vi "UHR-Fleezers Control (host) - Lorentz v5.vi"() -> ()   [LabVIEW 2014] (continued)
            n3482 = property on="All FB On/Off" class="Bool (strict)"("Val(Sgnl)"=FALSE) -> ()  [unwired: 2 in, 2 out]
          }
        }
      }
    }
    n3483 = flat-sequence "To save data" {
      tunnel: [w5298] -> w4515
      tunnel: [w5299] -> w4514
      tunnel: w4477 -> [w5292]
      tunnel: w4206 -> [w5296]
      tunnel: ["Save Calibration"] -> w4489
      tunnel: w4236 -> [w5295]
      tunnel: [w5288] -> w4486
      tunnel: [w5285] -> w4485
      tunnel: [w5282] -> w4484
      tunnel: w4476 -> [w5284]
      tunnel: w4172 -> [w5278]
      tunnel: [w5278] -> w4440
      tunnel: ["Start Saving"] -> w4420
      tunnel: [w5273] -> w4369
      tunnel: [w5272] -> w4368
      tunnel: [w5269] -> w4270
      tunnel: [w5265] -> w4258
      tunnel: w4515 -> [w5610]
      tunnel: w4514 -> [w5609]
      tunnel: w4237 -> [w5608]
      tunnel: w4489 -> [w5607]
      tunnel: w4486 -> [w5605]
      tunnel: w4485 -> [w5604]
      tunnel: w4484 -> [w5603]
      tunnel: w4229 -> [w5602]
      tunnel: w4235 -> [w5601]
      tunnel: w4440 -> [w5600]
      tunnel: w4420 -> [w5599]
      tunnel: w4277 -> [w5598]
      tunnel: w4319 -> [w5597]
      tunnel: w4369 -> [w5596]
      tunnel: w4368 -> [w5595]
      tunnel: w4367 -> [w5594]
      tunnel: w4178 -> [w5593]
      tunnel: w4234 -> [w5592]
      tunnel: w4270 -> [w5591]
      tunnel: w4258 -> [w5590]
      frame #0 {
        # "Changed by Ronen - we don't have a database so we disabled this"
        n3484 = Or(x="Save N Sets", y="Start Saving") -> (x .or. y?=w5279:bool)
        n3485 = To Double Precision Float(number=w5295) -> (double precision float=w5289:dbl)
        n3486 = Build Array(w5279, "Save Calibration", w5292, w5284, "Flow Cal") -> (w5294:bool[])
        n3487 = Compound Arithmetic op=OR("Save Calibration", w5292, w5279, w5284, "Flow Cal") -> (w5297:bool)
        n3488 = Boolean Array To Number(Boolean array=w5294) -> (number=w5291:u32)
        n3489 = feedback #21(FALSE ("Save APD Data\nwith Trap Data")) -> (w5274:bool)
        n3490 = feedback #22(refnum<k0> refnum) -> (w5300:refnum<file>)
        n3491 = feedback #23(FALSE ("Save APD Data\nwith Trap Data")) -> (w5283:bool)
        n3492 = feedback #24(0) -> (w5302:i32)
        n3493 = feedback #25() -> (w5290:u32)  [unwired: 1 out]
        n3494 = feedback #26(refnum<k0> refnum) -> (w5270:refnum<file>)
        n3495 = feedback #27(refnum<k0> refnum) -> (w5276:refnum<file>)
        n3496 = feedback #28(refnum<k0> refnum) -> (w5266:refnum<file>)
        n3497 = feedback #29(refnum<k0> refnum) -> (w5286:refnum<file>)
        n3498 = case shown="True" w5297 {
          tunnel: [w5311 1] -> w5298
          tunnel: w5302 -> [w5313 _]
          tunnel: [w5312 w5345] -> w5299
          tunnel: w5300 -> [w5312 _]
          tunnel: w5296 -> [_ w5363]
          tunnel: w5289 -> [_ w5361]
          tunnel: w5291 -> [_ w5364]
          tunnel: [w5310 w5344] -> w5288
          tunnel: w5290 -> [w5310 _]
          tunnel: [w5309 w5342] -> w5285
          tunnel: w5286 -> [w5309 _]
          tunnel: [w5308 w5341] -> w5282
          tunnel: w5283 -> [w5308 _]
          tunnel: "Start Saving" -> [_ w5339]
          tunnel: w5278 -> [_ w5338]
          tunnel: [w5307 w5331] -> w5272
          tunnel: w5276 -> [w5307 _]
          tunnel: [w5306 w5330] -> w5273
          tunnel: w5274 -> [w5306 _]
          tunnel: [w5305 w5316] -> w5269
          tunnel: w5270 -> [w5305 _]
          tunnel: [w5304 w5314] -> w5265
          tunnel: w5266 -> [w5304 _]
          frame False {
            n3499 = Increment(x=w5313) -> (x+1=w5311:i32)
          }
          frame True {
            w5315 = FALSE ("Start Saving")
            w5340 = 10.0  # File Version
            w5347 = FALSE ("prepend array or string size? (T)")
            w5346 = T44."big-endian, network order" ("byte order (0:big-endian, network order)")
            # "Ronen Changed the create file - changed data folder to c:\\Data"
            # "Save trap position\ndata"
            n3500 = Array Size(array=w5338) -> (size(s)=w5337:i32)
            n3501 = To Double Precision Float(number=w5337) -> (double precision float=w5336:dbl)
            n3502 = local read "BD 1 Frequency 1 (MHz)"() -> (w5360:dbl)
            n3503 = local read "BD 2 Frequency 1 (MHz)"() -> (w5359:dbl)
            n3504 = local read "BD 1 Frequency 2 (MHz)"() -> (w5358:dbl)
            n3505 = local read "BD 2 Frequency 2 (MHz)"() -> (w5357:dbl)
            n3506 = local read "BD 1 Frequency 3 (MHz)"() -> (w5356:dbl)
            n3507 = local read "BD 2 Frequency 3 (MHz)"() -> (w5355:dbl)
            n3508 = local write "Flow Cal"(w5315) -> ()
            n3509 = local write "Save Calibration"(w5315) -> ()
            n3510 = local write "Start Saving"(w5315) -> ()
            n3511 = Build Array("Save APD Data\nwith Trap Data", "Save Trap Pos. Data") -> (w5333:bool[])
            n3512 = Boolean Array To Number(Boolean array=w5333) -> (number=w5332:u32)
            n3513 = Build Array(w5360, w5359, w5358, w5357, w5356, w5355) -> (w5354:dbl[])
            n3514 = case shown="16" w5364 {
              tunnel: w5363 -> [w5464 w5491 w5507 w5545 w5582]
              tunnel: w5336 -> [w5469 w5498 w5527 w5564 w5587]
              tunnel: w5361 -> [w5468 w5497 w5526 w5563 w5586]
              tunnel: [w5465 w5493 w5518 w5555 w5583] -> w5352
              tunnel: [w5456 "Cal sets to save" w5508 w5546 w5569] -> w5344
              tunnel: w5354 -> [w5466 w5494 w5520 w5557 w5584]
              tunnel: "Save APD Data\nwith Trap Data" -> [w5463 w5480 w5504 w5543 w5581]
              tunnel: [w5463 w5478 w5504 w5543 w5581] -> w5341
              tunnel: w5340 -> [w5459 w5487 w5502 w5541 w5577]
              tunnel: w5339 -> [w5458 _ _ _ _]
              tunnel: [w5449 w5486 w5501 w5531 w5576] -> w5330
              tunnel: "Save Trap Pos. Data" -> [w5449 w5485 w5501 w5531 w5576]
              tunnel: w5332 -> [w5448 w5484 w5500 w5530 w5575]
              frame 1, Default {
                # "timeseries"
                n3515 = case shown="True" "Profile" {
                  tunnel: [w5472 w5476] -> w5453
                  tunnel: [w5472 w5475] -> w5452
                  tunnel: [w5472 w5474] -> w5451
                  tunnel: [w5472 w5473] -> w5450
                  frame False {
                    w5472 = 0.0 ("f")
                  }
                  frame True {
                    n3516 = local read "Current Position"() -> (w5477:cluster{dbl, dbl, dbl})
                    n3517 = local read "Y change (mm)"() -> (w5473:dbl)
                    n3518 = Unbundle(w5477) -> (w5476:dbl, w5475:dbl, w5474:dbl)
                  }
                }
                n3519 = local read "Save ave N"() -> (w5471:dbl)
                n3520 = Multiply(x=w5471, y=w5464) -> (x*y=w5470:dbl)
                n3521 = To Double Precision Float(number=w5448) -> (double precision float=w5462:dbl)
                n3522 = Build Array(w5459, w5464, w5470, w5469, w5468, 0.0 ("f")) -> (w5467:dbl[])
                n3523 = Build Array(w5462, w5453, w5452, w5451, w5450) -> (w5460:dbl[])
                n3524 = Select(t=u32 4000000000, s=w5458, f="N sets to save") -> (s? t:f=w5456:u32)
                n3525 = Build Array (concatenate)(w5467, w5466, w5460) -> (w5465:dbl[])
              }
              frame 2 {
                w5489 = 0.0 ("f")
                w5479 = FALSE ("Save APD Data\nwith Trap Data")
                # "For diagnostics save trap position\ndata during cal"
                # "calibration"
                n3526 = Boolean To (0,1)(Boolean=w5479) -> (0, 1=w5483:i16)
                n3527 = Select(t=w5480, s="Save trap pos with cal", f=w5479) -> (s? t:f=w5478:bool)
                n3528 = Select(t=w5485, s="Save trap pos with cal", f=w5479) -> (s? t:f=w5486:bool)
                n3529 = Select(t=w5484, s="Save trap pos with cal", f=w5483) -> (s? t:f=w5482:u32)
                n3530 = To Double Precision Float(number=w5482) -> (double precision float=w5490:dbl)
                n3531 = Build Array(w5487, w5491, w5491, w5498, w5497, 1.0 ("t")) -> (w5495:dbl[])
                n3532 = Build Array(w5490, w5489, w5489, w5489, w5489) -> (w5488:dbl[])
                n3533 = Build Array (concatenate)(w5495, w5494, w5488) -> (w5493:dbl[])
                "Calibrating Trap..." <- TRUE ("Calibrating...")
              }
              frame 4 {
                w5505 = 0.0 ("f")
                # "scan dir (x/y = 0/1)"
                # "cycles/step"
                # "n scans (f/b)"
                # "steps"
                # "freq. range"
                # "AOD raster scan"
                n3534 = local read "Number of F/B Scans (AOD)"() -> (w5512:u16)
                n3535 = local read "Cycles/step (AOD)"() -> (w5514:u64)
                n3536 = local read "Scan Range (MHz)"() -> (w5517:dbl)
                n3537 = local read "Scan steps (AOD)"() -> (w5516:u64)
                n3538 = local read "Scan BD"() -> (w5524:bool)
                n3539 = local read "Save ave N"() -> (w5529:dbl)
                n3540 = Boolean To (0,1)(Boolean=w5524) -> (0, 1=w5523:i16)
                n3541 = To Double Precision Float(number=w5512) -> (double precision float=w5511:dbl)
                n3542 = To Double Precision Float(number=w5516) -> (double precision float=w5515:dbl)
                n3543 = To Double Precision Float(number=w5514) -> (double precision float=w5513:dbl)
                n3544 = To Double Precision Float(number=w5523) -> (double precision float=w5522:dbl)
                n3545 = Multiply(x=w5529, y=w5507) -> (x*y=w5528:dbl)
                n3546 = To Double Precision Float(number=w5500) -> (double precision float=w5506:dbl)
                n3547 = Build Array(w5506, w5505, w5505, w5505, w5505) -> (w5503:dbl[])
                n3548 = local read "N sets should be saved"() -> (w5509:dbl)
                n3549 = Build Array(w5522, w5517, w5515, w5513, w5511) -> (w5519:dbl[])
                n3550 = Build Array(w5502, w5507, w5528, w5527, w5526, 2.0 ("t")) -> (w5521:dbl[])
                n3551 = Round Toward +Infinity(x=w5509) -> (ceil(x): smallest int >= x=w5510:dbl)
                n3552 = Build Array (concatenate)(w5521, w5520, w5503, w5519) -> (w5518:dbl[])
                n3553 = To Unsigned Long Integer(number=w5510) -> (unsigned 32bit integer=w5508:u32)
              }
              frame 8 {
                w5538 = 0.0 ("f")
                # "MCL raster scan"
                n3554 = local read "Number of scans (MCL)"() -> (w5533:u64)
                n3555 = local read "2D or 1D Scan"() -> (w5535:bool)
                n3556 = local read "Scan lines (y)"() -> (w5532:u64)
                n3557 = local read "Scan Range (V)\n(of steps)"() -> (w5554:dbl)
                n3558 = local read "Fast Scan Dir"() -> (w5561:bool)
                n3559 = local read "Cycles/step (MCL)"() -> (w5551:u64)
                n3560 = local read "Scan steps (MCL)"() -> (w5553:u64)
                n3561 = Select(t=w5532, s=w5535, f=w5533) -> (s? t:f=w5534:u64)
                n3562 = Boolean To (0,1)(Boolean=w5535) -> (0, 1=w5537:i16)
                n3563 = local read "Save ave N"() -> (w5566:dbl)
                n3564 = local read "Initial X"() -> (w5540:dbl)
                n3565 = local read "Initial Y"() -> (w5539:dbl)
                n3566 = To Double Precision Float(number=w5537) -> (double precision float=w5536:dbl)
                n3567 = Boolean To (0,1)(Boolean=w5561) -> (0, 1=w5560:i16)
                n3568 = To Double Precision Float(number=w5534) -> (double precision float=w5549:dbl)
                n3569 = To Double Precision Float(number=w5553) -> (double precision float=w5552:dbl)
                n3570 = To Double Precision Float(number=w5551) -> (double precision float=w5550:dbl)
                n3571 = To Double Precision Float(number=w5560) -> (double precision float=w5559:dbl)
                n3572 = Multiply(x=w5566, y=w5545) -> (x*y=w5565:dbl)
                n3573 = To Double Precision Float(number=w5530) -> (double precision float=w5544:dbl)
                n3574 = local read "N sets should be saved (MCL)"() -> (w5547:dbl)
                n3575 = Build Array(w5544, w5536, w5538, w5538, w5538) -> (w5542:dbl[])
                n3576 = Build Array(w5559, w5554, w5552, w5550, w5549, w5540, w5539) -> (w5556:dbl[])
                n3577 = Build Array(w5541, w5545, w5565, w5564, w5563, 3.0 ("t")) -> (w5558:dbl[])
                n3578 = Round Toward +Infinity(x=w5547) -> (ceil(x): smallest int >= x=w5548:dbl)
                n3579 = Build Array (concatenate)(w5558, w5557, w5542, w5556) -> (w5555:dbl[])
                n3580 = To Unsigned Long Integer(number=w5548) -> (unsigned 32bit integer=w5546:u32)
              }
              frame 16 {
                w5568 = 0.0
                # "Flow calibration - added by Ronen: Number\nof saved sets is distance (1 mm) divided by \nspeed +1.5 spare second divided by the time of\nset measurement, 0.2 sec for 2 set interlace"
                # "timeseries"
                n3581 = local read "Save ave N"() -> (w5589:dbl)
                n3582 = Reciprocal(x=0.0) -> (1/x=w5574:dbl)
                n3583 = Add(x=w5574, y=1.5) -> (x+y=w5572:dbl)
                n3584 = Multiply(x=w5589, y=w5582) -> (x*y=w5588:dbl)
                n3585 = Divide(x=w5572, y=0.2) -> (x/y=w5570:dbl)
                n3586 = To Double Precision Float(number=w5575) -> (double precision float=w5580:dbl)
                n3587 = To Unsigned Long Integer(number=w5570) -> (unsigned 32bit integer=w5569:u32)
                n3588 = Build Array(w5577, w5582, w5588, w5587, w5586, 4.0 ("f")) -> (w5585:dbl[])
                n3589 = Build Array(w5580, w5568, w5568, w5568, w5568) -> (w5578:dbl[])
                n3590 = Build Array (concatenate)(w5585, w5584, w5578) -> (w5583:dbl[])
              }
            }
            n3591 = local read "Index"() -> (w5369:dbl)
            n3592 = call "Create new save file.vi"("Insert"="", "Ext"=".dat", "Index In"=w5369) -> ("Path Out"=w5318:path, "Index Out"=w5343:dbl)
            n3593 = local write "Save file name"(w5318) -> ()
            n3594 = local write "Index"(w5343) -> ()
            n3595 = local write "Save index"(w5343) -> ()
            n3596 = case shown="True" "Save Event Log?" {
              tunnel: w5318 -> [_ w5383]
              tunnel: [refnum<k0> refnum w5382] -> w5316
              frame False {
              }
              frame True {
                (unwired) FALSE ("prepend array or string size? (T)")
                n3597 = Path To String(path=w5383) -> (string=w5394:string)
                n3598 = String Length(string=w5394) -> (length=w5393:i32)
                n3599 = Subtract(x=w5393, y=4) -> (x-y=w5391:i32)
                n3600 = String Subset(string=w5394, length (rest)=w5391) -> (substring=w5390:string)  [unwired: 1 out]
                n3601 = Concatenate Strings(w5390, "_log.txt" ("string")) -> (w5388:string)
                n3602 = String To Path(string=w5388) -> (path=w5384:path)
                n3603 = Open/Create/Replace File(file path (use dialog)=w5384, operation (0:open)=T43."create", access (0:read/write)=enum16{"read/write", "read-only", "write-only"}."write-only") -> (refnum out=w5385:refnum<file>)  [unwired: 1 in, 4 out]
                n3604 = Deny Access(7:w5385) -> (3:w5382:refnum<file>)  [unwired: 1 in, 2 out]
                n3605 = call "write to event log.vi"("log file ref"=w5382, "time"=0.0, "input string"="start log") -> ()  [unwired: 8 in]
              }
            }
            "log file ref" <- w5316
            n3606 = Array Size(array=w5352) -> (size(s)=w5353:i32)
            n3607 = Open/Create/Replace File(file path (use dialog)=w5318, operation (0:open)=T43."create", access (0:read/write)=enum16{"read/write", "read-only", "write-only"}."write-only") -> (refnum out=w5366:refnum<file>)  [unwired: 1 in, 4 out]
            n3608 = local write "Saving..."(TRUE ("Saving...")) -> ()
            n3609 = To Double Precision Float(number=w5353) -> (double precision float=w5351:dbl)
            n3610 = String Length(string="Comment (data description)") -> (length=w5350:i32)
            n3611 = To Double Precision Float(number=w5350) -> (double precision float=w5349:dbl)
            n3612 = Deny Access(7:w5366) -> (3:w5365:refnum<file>)  [unwired: 1 in, 2 out]
            n3613 = Build Array (concatenate)(w5351, w5352, w5349) -> (w5328:dbl[])
            n3614 = case "If fluorescence data to be saved" shown="True" w5341 {
              tunnel: w5318 -> [_ w5447]
              tunnel: [w5417 w5430] -> w5342
              tunnel: [w5417 w5418] -> w5314
              frame False {
                w5417 = refnum<k0> refnum
              }
              frame True {
                w5429 = 0.0
                w5422 = T43."create" ("operation (0:open)")
                w5423 = enum16{"read/write", "read-only", "write-only"}."write-only" ("access (0:read/write)")
                n3615 = local read "APD Integration Time (s)"() -> (w5435:dbl)
                n3616 = local read "N APD Samp/step"() -> (w5428:dbl)
                n3617 = local read "Number of APDs"() -> (w5427:u8)
                n3618 = Path To String(path=w5447) -> (string=w5446:string)
                n3619 = String Length(string=w5446) -> (length=w5445:i32)
                n3620 = Subtract(x=w5445, y=4) -> (x-y=w5443:i32)
                n3621 = String Subset(string=w5446, length (rest)=w5443) -> (substring=w5426:string)  [unwired: 1 out]
                n3622 = Build Array(w5435, w5428, w5427, w5429, w5429, w5429, w5429, w5429) -> (w5432:dbl[])
                n3623 = Concatenate Strings(w5426, "_green.dat") -> (w5424:string)
                n3624 = Concatenate Strings(w5426, "_fl.dat" ("string")) -> (w5441:string)
                n3625 = Array Size(array=w5432) -> (size(s)=w5434:i32)
                n3626 = String To Path(string=w5441) -> (path=w5439:path)
                n3627 = Open/Create/Replace File(file path (use dialog)=w5439, operation (0:open)=w5422, access (0:read/write)=w5423) -> (refnum out=w5440:refnum<file>)  [unwired: 1 in, 4 out]
                n3628 = Deny Access(7:w5440) -> (3:w5436:refnum<file>)  [unwired: 1 in, 2 out]
                n3629 = String To Path(string=w5424) -> (path=w5421:path)
                n3630 = To Double Precision Float(number=w5434) -> (double precision float=w5433:dbl)
                n3631 = Build Array (concatenate)(w5433, w5432) -> (w5431:dbl[])
                n3632 = Write to Binary File(file (use dialog)=w5436, data=w5431, 5:FALSE ("prepend array or string size? (T)"), 9:T44."big-endian, network order" ("byte order (0:big-endian, network order)")) -> (refnum out=w5430:refnum<file>)  [unwired: 1 in, 3 out]
                n3633 = Open/Create/Replace File(file path (use dialog)=w5421, operation (0:open)=w5422, access (0:read/write)=w5423) -> (refnum out=w5419:refnum<file>, error out=w5420:errorcluster)  [unwired: 3 in, 1 out]
                n3634 = Deny Access(4:w5420, 7:w5419) -> (3:w5418:refnum<file>)  [unwired: 1 in, 1 out]
              }
            }
            n3635 = case shown="True" w5330 {
              tunnel: w5318 -> [_ w5402]
              tunnel: [refnum<k0> refnum w5401] -> w5331
              frame False {
              }
              frame True {
                w5397 = 0.0 ("element")
                n3636 = Path To String(path=w5402) -> (string=w5416:string)
                n3637 = Build Array(w5397, w5397, w5397, w5397, w5397, w5397, w5397, w5397) -> (w5398:dbl[])
                n3638 = String Length(string=w5416) -> (length=w5415:i32)
                n3639 = Subtract(x=w5415, y=4) -> (x-y=w5413:i32)
                n3640 = Array Size(array=w5398) -> (size(s)=w5400:i32)
                n3641 = String Subset(string=w5416, length (rest)=w5413) -> (substring=w5412:string)  [unwired: 1 out]
                n3642 = To Double Precision Float(number=w5400) -> (double precision float=w5399:dbl)
                n3643 = Concatenate Strings(w5412, "_pos.dat" ("string")) -> (w5410:string)
                n3644 = Build Array (concatenate)(w5399, w5398) -> (w5396:dbl[])
                n3645 = String To Path(string=w5410) -> (path=w5406:path)
                n3646 = Open/Create/Replace File(file path (use dialog)=w5406, operation (0:open)=T43."create", access (0:read/write)=enum16{"read/write", "read-only", "write-only"}."write-only") -> (refnum out=w5407:refnum<file>)  [unwired: 1 in, 4 out]
                n3647 = Deny Access(7:w5407) -> (3:w5403:refnum<file>)  [unwired: 1 in, 2 out]
                n3648 = Write to Binary File(file (use dialog)=w5403, data=w5396, 5:FALSE ("prepend array or string size? (T)"), 9:T44."big-endian, network order" ("byte order (0:big-endian, network order)")) -> (refnum out=w5401:refnum<file>)  [unwired: 1 in, 3 out]
              }
            }
            n3649 = Write to Binary File(file (use dialog)=w5365, data=w5328, 5:w5347, 9:w5346) -> (refnum out=w5348:refnum<file>)  [unwired: 1 in, 3 out]
            n3650 = Write to Binary File(file (use dialog)=w5348, data="Comment (data description)", 5:w5347, 9:w5346) -> (refnum out=w5345:refnum<file>)  [unwired: 1 in, 3 out]
            n3651 = local read "connection reference"() -> (w5329:T24)
            n3652 = Bundle("Comment (data description)"="Comment (data description)", "Channel 1 Buffer"="Channel 1 Buffer", "Channel 2 Buffer"="Channel 2 Buffer", "Channel 3 Buffer"="Channel 3 Buffer", "Title"="Title", "DNA Construct"="DNA Construct", "Bead diameter"="Bead diameter", "Name"="Name") -> (w5319:T63)  [unwired: 1 in]
            n3653 = disable-structure shown="Disabled" {
              disable-tunnel: w5329 -> [w5377 _]
              disable-tunnel: w5328 -> [w5375 _]
              disable-tunnel: w5319 -> [w5374 _]
              disable-tunnel: w5318 -> [w5373 _]
              frame Disabled {
                n3654 = call "MattFileCreator-v9.vi"("Comments"=w5374, "Input Array"=w5375, "File path"=w5373, "table"="labview", "connection reference"=w5377) -> ("connection reference out"=w5376:T24)  [unwired: 5 in, 1 out]
                n3655 = local write "connection reference"(w5376) -> ()
              }
              frame Enabled {
              }
            }
          }
        }
        n3656 = feedback-in #21(w5273) -> ()
        n3657 = feedback-in #22(w5299) -> ()
        n3658 = feedback-in #23(w5282) -> ()
        n3659 = feedback-in #24(w5298) -> ()
        n3660 = feedback-in #25(w5288) -> ()
        n3661 = feedback-in #26(w5269) -> ()
        n3662 = feedback-in #27(w5272) -> ()
        n3663 = feedback-in #28(w5265) -> ()
        n3664 = feedback-in #29(w5285) -> ()
      }
      frame #1 {
        n3665 = local read "Saving..."() -> (w5606:bool)
        n3666 = case shown="True" w5606 {
          tunnel: w5610 -> [_ w5624]
          tunnel: w5609 -> [_ w5638]
          tunnel: w5608 -> [_ w5634]
          tunnel: w5607 -> [_ w5633]
          tunnel: w5605 -> [_ w5632]
          tunnel: w5604 -> [_ w5627]
          tunnel: w5603 -> [_ w5626]
          tunnel: w5602 -> [_ w5625]
          tunnel: w5601 -> [_ w5623]
          tunnel: w5600 -> [_ w5621]
          tunnel: w5599 -> [_ w5620]
          tunnel: w5598 -> [_ w5619]
          tunnel: w5597 -> [_ w5618]
          tunnel: w5596 -> [_ w5617]
          tunnel: w5595 -> [_ w5616]
          tunnel: w5594 -> [_ w5615]
          tunnel: w5593 -> [_ w5614]
          tunnel: w5592 -> [_ w5613]
          tunnel: w5591 -> [_ w5612]
          tunnel: w5590 -> [_ w5611]
          frame False {
          }
          frame True {
            n3667 = Multiply(x=w5624, y=w5623) -> (x*y=→"Time (s)":dbl)
            n3668 = Less Or Equal?(x=w5624, y=w5632) -> (x <= y?=w5636:bool)
            n3669 = Compound Arithmetic op=OR("Stop Saving", "Abort save 2") -> (w5628:bool)
            n3670 = Not(x=w5628) -> (.not. x?=w5637:bool)
            n3671 = And(x=w5636, y=w5637) -> (x .and. y?=w5635:bool)
            n3672 = case shown="True" w5635 {
              tunnel: w5638 -> [w5648 w5749]
              tunnel: [0.0 w5752] -> w5631
              tunnel: w5624 -> [_ w5750]
              tunnel: w5632 -> [_ w5751]
              tunnel: w5634 -> [_ w5746]
              tunnel: w5633 -> [_ _]
              tunnel: w5627 -> [w5646 w5739]
              tunnel: w5626 -> [w5645 w5740]
              tunnel: w5625 -> [_ w5738]
              tunnel: w5621 -> [_ w5737]
              tunnel: w5620 -> [_ w5655]
              tunnel: w5619 -> [_ w5730]
              tunnel: w5618 -> [_ w5677]
              tunnel: w5617 -> [w5642 w5694]
              tunnel: w5616 -> [w5643 w5693]
              tunnel: w5615 -> [_ w5690]
              tunnel: w5614 -> [_ w5688]
              tunnel: w5613 -> [_ w5654]
              tunnel: w5612 -> [w5641 _]
              tunnel: w5611 -> [w5639 w5653]
              frame False {
                w5644 = FALSE
                n3673 = Close File(refnum=w5648) -> ()  [unwired: 1 in, 2 out]
                n3674 = case shown="True" w5645 {
                  tunnel: w5646 -> [_ w5652]
                  tunnel: w5639 -> [_ w5651]
                  frame False {
                  }
                  frame True {
                    n3675 = Close File(refnum=w5652) -> ()  [unwired: 1 in, 2 out]
                    n3676 = Close File(refnum=w5651) -> ()  [unwired: 1 in, 2 out]
                  }
                }
                n3677 = case shown="True" w5642 {
                  tunnel: w5643 -> [_ w5650]
                  frame False {
                  }
                  frame True {
                    n3678 = Close File(refnum=w5650) -> ()  [unwired: 1 in, 2 out]
                  }
                }
                n3679 = local read "Save Event Log?"() -> (w5640:bool)
                n3680 = case shown="True" w5640 {
                  tunnel: w5641 -> [_ w5649]
                  frame False {
                  }
                  frame True {
                    n3681 = Close File(refnum=w5649) -> ()  [unwired: 1 in, 2 out]
                  }
                }
                n3682 = local write "Raster Scanning..."(w5644) -> ()
                n3683 = local write "Calibrating Trap..."(w5644) -> ()
                n3684 = call <vilib>:"Beep.vi"() -> ()  [unwired: 3 in, 9 out]
                n3685 = local write "Stop Saving"(w5644) -> ()
                "Saving..." <- w5644
              }
              frame True {
                n3686 = local read "Calibrating Trap..."() -> (w5741:bool)
                n3687 = case "Write fl. data" shown="True" w5740 {
                  tunnel: w5739 -> [_ w5782]
                  tunnel: w5738 -> [_ w5781]
                  tunnel: w5653 -> [_ w5775]
                  frame False {
                  }
                  frame True {
                    w5774 = FALSE ("prepend array or string size? (T)")
                    w5776 = T44."big-endian, network order" ("byte order (0:big-endian, network order)")
                    n3688 = property on="Green Laser ON" class="Bool (strict)"() -> ("Value"=w5780:bool)  [unwired: 2 in, 2 out]
                    n3689 = property on="Green Intensity % (FB OFF)" class="DigNum (strict)"() -> ("Value"=w5779:dbl)  [unwired: 2 in, 2 out]
                    n3690 = Boolean To (0,1)(Boolean=w5780) -> (0, 1=w5778:i16)
                    n3691 = Multiply(x=w5778, y=w5779) -> (x*y=w5777:dbl)
                    n3692 = Write to Binary File(file (use dialog)=w5782, data=w5781, 5:w5774, 9:w5776) -> ()  [unwired: 1 in, 4 out]
                    n3693 = Write to Binary File(file (use dialog)=w5775, data=w5777, 5:w5774, 9:w5776) -> ()  [unwired: 2 in, 3 out]
                  }
                }
                n3694 = Greater?(x="Save ave N", y=1.0) -> (0:w5744:bool)
                n3695 = Not(x=w5741) -> (.not. x?=w5743:bool)
                n3696 = And(x=w5743, y=w5744) -> (x .and. y?=w5691:bool)
                n3697 = case shown="True" w5691 {
                  tunnel: w5690 -> [w5755 w5766]
                  tunnel: [w5755 w5758] -> w5689
                  tunnel: "Save ave N" -> [_ w5759]
                  frame False {
                  }
                  frame True {
                    w5756 = 2 ("dimension size")
                    n3698 = Array Size(array=w5766) -> (size(s)=w5760:i32)
                    n3699 = Divide(x=w5760, y=w5756) -> (x/y=w5764:dbl)
                    n3700 = Reshape Array(w5766, w5764, w5756) -> (w5765:u64[][])
                    n3701 = Transpose 2D Array(2D array=w5765) -> (transposed array=w5763:u64[][])
                    n3702 = for {
                      tunnel: w5763 -> [w5768] mode=indexing
                      tunnel: [w5767] -> w5757 mode=indexing
                      tunnel: w5759 -> [w5769]
                      workers-P: _ -> [_]
                      n3703 = call "downsample 1D array - U64.vi"("Ave N"=w5769, "Array In"=w5768) -> ("Array Out"=w5767:u64[])  [unwired: 1 in]
                    }
                    n3704 = Transpose 2D Array(2D array=w5757) -> (transposed array=w5762:u64[][])
                    n3705 = Divide(x=w5760, y=w5759) -> (x/y=w5761:dbl)
                    n3706 = Reshape Array(w5762, w5761) -> (w5758:u64[])
                  }
                }
                n3707 = case shown="True" w5691 {
                  tunnel: w5746 -> [w5783 w5795]
                  tunnel: [w5783 w5787] -> w5742
                  tunnel: "Save ave N" -> [_ w5788]
                  tunnel: w5737 -> [_ w5786]
                  frame False {
                  }
                  frame True {
                    n3708 = Array Size(array=w5795) -> (size(s)=w5789:i32)
                    n3709 = Array Size(array=w5786) -> (size(s)=w5785:i32)
                    n3710 = Divide(x=w5789, y=w5785) -> (x/y=w5793:dbl)
                    n3711 = Reshape Array(w5795, w5793, w5785) -> (w5794:i16[][])
                    n3712 = Transpose 2D Array(2D array=w5794) -> (transposed array=w5792:i16[][])
                    n3713 = for {
                      tunnel: w5792 -> [w5798] mode=indexing
                      tunnel: [w5797] -> w5784 mode=indexing
                      tunnel: w5788 -> [w5796]
                      workers-P: _ -> [_]
                      n3714 = call "downsample 1D array - I16 to F32.vi"("Ave N"=w5796, "Array In"=w5798) -> ("Array Out"=w5797:sgl[])  [unwired: 1 in]
                    }
                    n3715 = Transpose 2D Array(2D array=w5784) -> (transposed array=w5791:sgl[][])
                    n3716 = Divide(x=w5789, y=w5788) -> (x/y=w5790:dbl)
                    n3717 = Reshape Array(w5791, w5790) -> (w5787:sgl[])
                  }
                }
                n3718 = Index Array(array=w5677, index=2) -> (element=w5678:waveform(dbl))
                n3719 = Index Array(array=w5677, index=1) -> (element=w5711:waveform(dbl))
                n3720 = Index Array(array=w5677, index=0) -> (element=w5713:waveform(dbl))
                n3721 = Unbundle By Name(w5678) -> ("Y"=w5680:dbl[])
                n3722 = Unbundle By Name(w5711) -> ("Y"=w5715:dbl[])
                n3723 = Unbundle By Name(w5713) -> ("Y"=w5723:dbl[])
                n3724 = case "Write trap pos. data" shown="True" w5694 {
                  tunnel: w5693 -> [_ w5771]
                  tunnel: w5689 -> [_ w5770]
                  frame False {
                  }
                  frame True {
                    n3725 = Write to Binary File(file (use dialog)=w5771, data=w5770, 5:FALSE ("prepend array or string size? (T)"), 9:T44."big-endian, network order" ("byte order (0:big-endian, network order)")) -> ()  [unwired: 1 in, 4 out]
                  }
                }
                n3726 = Write to Binary File(file (use dialog)=w5749, data=w5742, 5:FALSE ("prepend array or string size? (T)"), 9:T44."big-endian, network order" ("byte order (0:big-endian, network order)")) -> ()  [unwired: 1 in, 4 out]
                n3727 = feedback #30(w5680) -> (w5681:dbl[])
                n3728 = Build Array (concatenate)(w5681, w5680) -> (w5676:dbl[])
                n3729 = Select(t=w5680, s=w5655, f=w5676) -> (s? t:f=w5666:dbl[])
                n3730 = feedback-in #30(w5666) -> ()
                n3731 = feedback #31(w5715) -> (w5717:dbl[])
                n3732 = Build Array (concatenate)(w5717, w5715) -> (w5716:dbl[])
                n3733 = Select(t=w5715, s=w5655, f=w5716) -> (s? t:f=w5705:dbl[])
                n3734 = feedback-in #31(w5705) -> ()
                n3735 = feedback #32(w5723) -> (w5736:dbl[])
                n3736 = Build Array (concatenate)(w5736, w5723) -> (w5735:dbl[])
                n3737 = Select(t=w5723, s=w5655, f=w5735) -> (s? t:f=w5710:dbl[])
                n3738 = feedback-in #32(w5710) -> ()
                n3739 = Divide(x=w5750, y=w5751) -> (x/y=w5753:dbl)
                n3740 = Multiply(x=w5753, y=100.0) -> (x*y=w5752:dbl)
                n3741 = Build Array(w5710, w5705, w5666) -> (→"Saved APD":dbl[][])
                n3742 = Array Size(array=w5710) -> (size(s)=w5728:i32)
                n3743 = Unbundle By Name(w5730) -> ("Y"=w5734:dbl[])
                n3744 = Subtract(x=w5728, y="N pts to average") -> (x-y=w5663:i32)
                n3745 = Multiply(x="N pts to average", y=u16 2) -> (x*y=w5706:u16)
                n3746 = Subtract(x=w5728, y=w5706) -> (x-y=w5664:i32)
                n3747 = feedback #33(w5734) -> (w5733:dbl[])
                n3748 = Build Array (concatenate)(w5733, w5734) -> (w5732:dbl[])
                n3749 = Select(t=w5734, s=w5655, f=w5732) -> (s? t:f=w5731:dbl[])
                "Trap Delta Graph" <- w5731
                n3750 = feedback-in #33(w5731) -> ()
                n3751 = Array Subset(array=w5710, index=w5663, length="N pts to average") -> (w5727:dbl[])
                n3752 = Array Subset(array=w5710, index=w5664, length="N pts to average") -> (w5726:dbl[])
                n3753 = Array Subset(array=w5705, index=w5663, length="N pts to average") -> (w5708:dbl[])
                n3754 = Array Subset(array=w5705, index=w5664, length="N pts to average") -> (w5707:dbl[])
                n3755 = Array Subset(array=w5666, index=w5663, length="N pts to average") -> (w5675:dbl[])
                n3756 = Array Subset(array=w5666, index=w5664, length="N pts to average") -> (w5674:dbl[])
                n3757 = Index Array(array=w5688, index=0) -> (element=w5686:waveform(dbl))
                n3758 = call-poly <vilib>:"Mean.vi"("X"=w5727) -> ("mean"=w5725:dbl)  [unwired: 1 out]
                n3759 = call-poly <vilib>:"Mean.vi"("X"=w5708) -> ("mean"=w5704:dbl)  [unwired: 1 out]
                n3760 = call-poly <vilib>:"Mean.vi"("X"=w5726) -> ("mean"=w5724:dbl)  [unwired: 1 out]
                n3761 = call-poly <vilib>:"Mean.vi"("X"=w5707) -> ("mean"=w5703:dbl)  [unwired: 1 out]
                n3762 = call-poly <vilib>:"Mean.vi"("X"=w5675) -> ("mean"=w5673:dbl)  [unwired: 1 out]
                n3763 = call-poly <vilib>:"Mean.vi"("X"=w5674) -> ("mean"=w5672:dbl)  [unwired: 1 out]
                n3764 = Unbundle By Name(w5686) -> ("Y"=w5684:dbl[])
                n3765 = Subtract(x=w5704, y=w5703) -> (x-y=w5695:dbl)
                "Delta Fl. 2" <- w5695
                n3766 = Subtract(x=w5673, y=w5672) -> (x-y=w5667:dbl)
                "Delta Fl. 3" <- w5667
                n3767 = Subtract(x=w5725, y=w5724) -> (x-y=w5722:dbl)
                "Delta Fl. 1" <- w5722
                n3768 = feedback #34(w5684) -> (w5683:dbl[])
                n3769 = Build Array (concatenate)(w5683, w5684) -> (w5685:dbl[])
                n3770 = Initialize Array(w5722, 1 ("dimension size")) -> (w5719:dbl[])
                n3771 = Initialize Array(w5695, 1 ("dimension size")) -> (w5700:dbl[])
                n3772 = Initialize Array(w5667, 1 ("dimension size")) -> (w5669:dbl[])
                n3773 = Select(t=w5684, s=w5655, f=w5685) -> (s? t:f=w5682:dbl[])
                "Saved trap pos" <- w5682
                n3774 = feedback-in #34(w5682) -> ()
                n3775 = feedback #35(w5719) -> (w5720:dbl[])
                n3776 = Build Array (concatenate)(w5720, w5719) -> (w5718:dbl[])
                n3777 = feedback #36(w5700) -> (w5701:dbl[])
                n3778 = feedback #37(w5669) -> (w5670:dbl[])
                n3779 = Build Array (concatenate)(w5701, w5700) -> (w5699:dbl[])
                n3780 = Build Array (concatenate)(w5670, w5669) -> (w5668:dbl[])
                n3781 = Select(t=w5719, s=w5655, f=w5718) -> (s? t:f=w5698:dbl[])
                n3782 = feedback-in #35(w5698) -> ()
                n3783 = Select(t=w5700, s=w5655, f=w5699) -> (s? t:f=w5697:dbl[])
                n3784 = feedback-in #36(w5697) -> ()
                n3785 = Select(t=w5669, s=w5655, f=w5668) -> (s? t:f=w5662:dbl[])
                n3786 = feedback-in #37(w5662) -> ()
                n3787 = Build Array(w5698, w5697, w5662) -> (→"Save APD Deriv":dbl[][])
                n3788 = Index Array(array=w5654, index=15) -> (element=w5660:waveform(dbl))
                n3789 = Unbundle By Name(w5660) -> ("Y"=w5658:dbl[])
                n3790 = feedback #38(w5658) -> (w5657:dbl[])
                n3791 = Build Array (concatenate)(w5657, w5658) -> (w5659:dbl[])
                n3792 = Select(t=w5658, s=w5655, f=w5659) -> (s? t:f=w5656:dbl[])
                "Amp current" <- w5656
                n3793 = feedback-in #38(w5656) -> ()
              }
            }
            "Progress" <- w5631
            "Progress 2" <- w5631
          }
        }
      }
    }
    n3794 = local read "wait to reset values"() -> (w4499:bool)
    n3795 = Not(x=w4497) -> (.not. x?=w4500:bool)
    n3796 = And(x=w4500, y=w4499) -> (x .and. y?=w4501:bool)
    n3797 = case "Part of MCL raster scanning: returns to initial positions after scan done" shown="True" w4501 {
      tunnel: w4247 -> [w5094 w5101]
      tunnel: [w5094 w5100] -> w4503
      tunnel: w4348 -> [w5093 w5099]
      tunnel: [w5093 w5098] -> w4498
      frame False {
      }
      frame True {
        w5109 = 10.0 ("y")
        w5108 = 32767.0 ("y")
        # "to return scan values\nafter a synchronous \nAOM scan"
        n3798 = local read "AO2"() -> (w5102:dbl)
        n3799 = local read "AO1"() -> (w5103:dbl)
        n3800 = local write "wait to reset values"(FALSE ("wait to reset values")) -> ()
        n3801 = Multiply(x=w5103, y=w5108) -> (x*y=w5105:dbl)
        n3802 = Multiply(x=w5102, y=w5108) -> (x*y=w5107:dbl)
        n3803 = Divide(x=w5105, y=w5109) -> (x/y=w5104:dbl)
        n3804 = Divide(x=w5107, y=w5109) -> (x/y=w5106:dbl)
        n3805 = To Word Integer(number=w5104) -> (16bit integer=w5110:i16)
        n3806 = To Word Integer(number=w5106) -> (16bit integer=w5111:i16)
        n3807 = local read "Total Counts (ticks)"() -> (w5095:u16)
        n3808 = local read "Scan Range (V)\n(of steps)"() -> (w5096:dbl)
        n3809 = xnode "Read/Write Control"("FPGA VI Reference In"=w5101, "error in"=w5099, "AO1"=w5110, "AO2"=w5111, "MCL count"=w5095) -> ("FPGA VI Reference Out"=w5100:T35, "error out"=w5098:errorcluster)
        n3810 = property on="Scan Range (V)\n(of steps)" class="DigNum (strict)"("Val(Sgnl)"=w5096) -> ()  [unwired: 2 in, 2 out]
      }
    }
    n3811 = case shown="True" "Sound ON" {
      tunnel: [w4614 w4659] -> w4300
      tunnel: w4299 -> [w4614 w4658]
      tunnel: w4297 -> [_ _]
      tunnel: w4276 -> [_ w4617]
      tunnel: w4296 -> [_ _]
      tunnel: w4295 -> [_ w4628]
      tunnel: w4294 -> [_ w4638]
      frame False {
      }
      frame True {
        n3812 = Index Array(array=w4617, index="Data channel to sound") -> (element=w4616:waveform(dbl))
        "Waveform Graph 2" <- w4616
        n3813 = Unbundle By Name(w4616) -> ("dt"=w4642:dbl, "Y"=w4640:dbl[])
        n3814 = Array Size(array=w4640) -> (size(s)=w4641:i32)
        "N data samples" <- w4641
        n3815 = for "Data time base" {
          N: w4641 -> [_]
          tunnel: [w4663] -> w4643 mode=indexing
          i -> [w4663]
        }
        n3816 = Multiply(x=w4642, y=w4643) -> (x*y=w4639:dbl[])
        n3817 = Compound Arithmetic op=MULTIPLY(6.283185307179586, "Carrier Frequency (Hz)", w4638) -> (w4655:dbl[])
        n3818 = call <vilib>:"Interpolate 1D.vi"("X is monotonic"=TRUE, "xi"=w4638, "X"=w4639, "Y"=w4640) -> ("yi"=w4636:dbl[])  [unwired: 5 in, 2 out]
        n3819 = Sine(x=w4655) -> (sin(x)=w4644:dbl[])
        n3820 = Add(x=w4636, y="Offset") -> (x+y=w4634:dbl[])
        n3821 = Multiply(x=w4634, y="mult x") -> (x*y=w4632:dbl[])
        n3822 = Add(x="Offset 2", y=w4632) -> (x+y=w4627:dbl[])
        n3823 = Compound Arithmetic op=MULTIPLY(6.283185307179586, "Carrier Frequency (Hz)", w4628, w4627) -> (w4619:dbl[])
        n3824 = for "Cumulative sum" {
          tunnel: [w4662] -> w4625 mode=indexing
          shift-right: [w4662] -> w4622
          shift-left: 0.0 -> [w4661]
          tunnel: w4619 -> [w4660] mode=indexing
          n3825 = Add(x=w4660, y=w4661) -> (x+y=w4662:dbl)
        }
        n3826 = feedback #39(0.0) -> (w4621:dbl)
        n3827 = Add(x=w4625, y=w4621) -> (x+y=w4624:dbl[])
        n3828 = Add(x=w4622, y=w4621) -> (x+y=w4620:dbl)
        n3829 = feedback-in #39(w4620) -> ()
        n3830 = Sine(x=w4624) -> (sin(x)=w4618:dbl[])
        n3831 = Select(t=w4644, s="tone or data", f=w4618) -> (s? t:f=w4650:dbl[])
        n3832 = Multiply(x=w4650, y="Volume") -> (x*y=w4648:dbl[])
        n3833 = Initialize Array(0.0 ("element"), "N initial buffer elements") -> (w4651:dbl[])
        n3834 = Multiply(x="N initial buffer elements", y=w4628) -> (x*y=→"Initial buffer time (s)":dbl)
        n3835 = Build Array (concatenate)(w4651, w4648) -> (w4653:dbl[])
        n3836 = First Call?() -> (First Call?: T/F=w4654:bool)
        n3837 = Select(t=w4653, s=w4654, f=w4648) -> (s? t:f=w4647:dbl[])
        n3838 = call-poly <vilib>:"Sound Output Write.vi"("data"=w4647, "task ID"=w4658) -> ("task ID out"=w4659:T50)  [unwired: 8 in, 1 out]
      }
    }
    n3839 = node-c288() -> ()  [unwired: 2 out]
  }
  n3840 = disable-structure shown="Disabled" {
    disable-tunnel: w16 -> [w5799 _]
    frame Disabled {
      n3841 = call <vilib>:"Sound Output Clear.vi"("task ID"=w5799) -> ()  [unwired: 10 in, 1 out]
    }
    frame Enabled {
    }
  }
  n3842 = node-c288(w59) -> ()  [unwired: 1 out]
  n3843 = node-c288(w67) -> ()  [unwired: 1 out]
  n3844 = flat-sequence {
    tunnel: w74 -> [w5803]
    tunnel: w75 -> [w5804]
    tunnel: [w5802] -> w73
    tunnel: [w5801] -> w72
    tunnel: w71 -> [_]
    tunnel: w69 -> [_]
    tunnel: w65 -> [_]
    tunnel: w73 -> [w5805]
    tunnel: w72 -> [w5806]
    frame #0 {
      w5800 = FALSE ("AI to FIFO")
      n3845 = xnode "Read/Write Control"("FPGA VI Reference In"=w5804, "error in"=w5803, "AI to FIFO"=w5800, "APD to FIFO"=w5800) -> ("FPGA VI Reference Out"=w5802:T35, "error out"=w5801:errorcluster)
    }
    frame #1 {
      n3846 = xnode "Close FPGA VI Reference"("FPGA VI Reference In"=w5805, "error in"=w5806) -> ("error out"=→"error out":errorcluster)
    }
  }
